vi "Application_CreateUninstallerBat.vi"(7 "TemporaryBatLocation":T1 items=["User Home"=0, "User Desktop"=1, "User Documents"=2, "User Application Data"=3, "User Preferences"=4, "User Temporary"=5, "Public Documents"=6, "Public Application Data"=7, "Public Preferences"=8, "Public Cache"=13, "System Core Libraries"=9, "System Installed Libraries"=10, "Application Files"=11, "Boot Volume Root"=12], 8 "error in":errorcluster, 11 "Project Name":string="BioReactor.lvproj") -> (0 "error IO":errorcluster)   [LabVIEW 2016]
doc: "Creates a windows .bat file with a time delay which is going to restart the project.\n\nAndreas Elmiger, 16.01.2017"
uses:
  <vilib>/Utility/sysdir.llb/System Directory Type.ctl
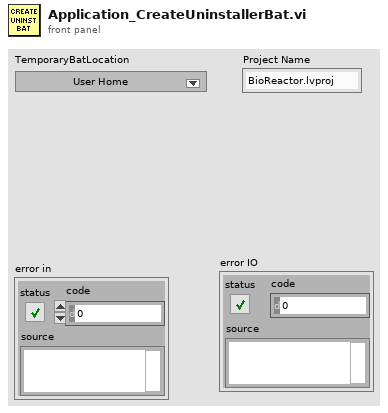
[diagram p1: front panel]
types:
  T1 = typedef "System Directory Type.ctl" = i32
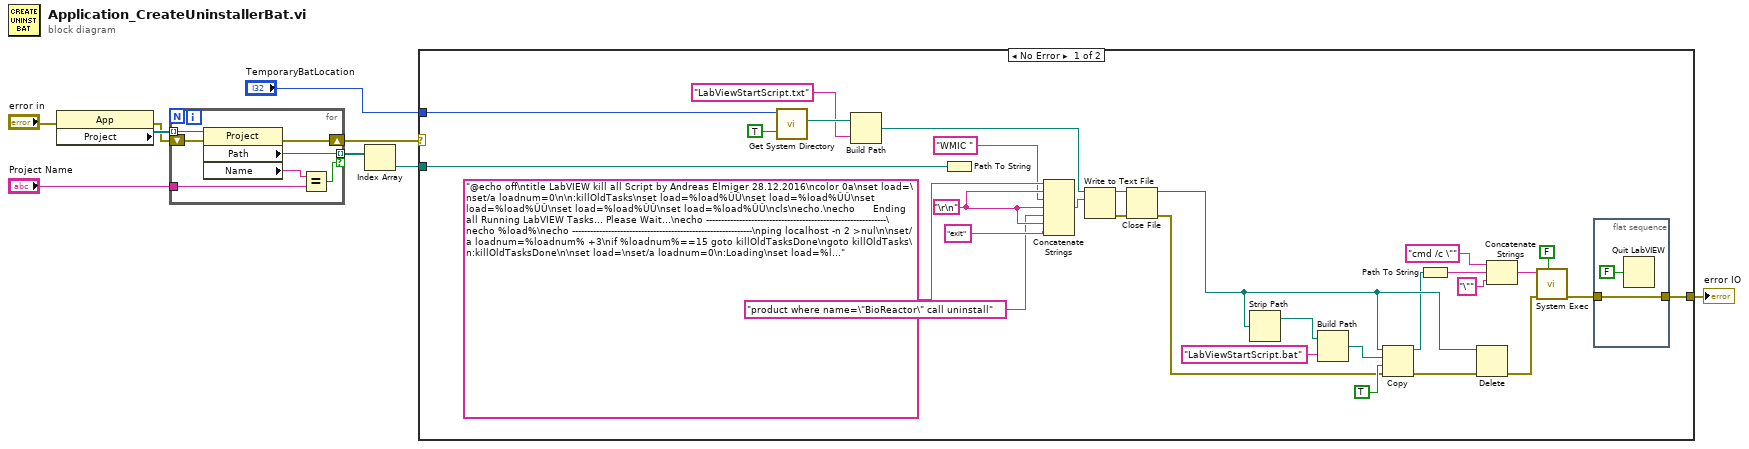
[diagram p0: block diagram]
diagram:
  n1 = property class="App"(error in="error in") -> (error out=w2:errorcluster, "Project"=w7:refnum<vi>[])  [unwired: 1 in, 1 out]
  n2 = for {
    tunnel: w7 -> [w16] mode=indexing
    tunnel: [w15] -> w5 mode=indexing if=w12
    tunnel: "Project Name" -> [w13]
    shift-right: [w10] -> w1
    shift-left: w2 -> [w11]
    n3 = property class="Project"(reference=w16, error in=w11) -> (error out=w10:errorcluster, "Path"=w15:path, "Name"=w14:string)  [unwired: 1 out]
    n4 = Equal?(x=w14, y=w13) -> (x = y?=w12:bool)
  }
  n5 = Index Array(array=w5) -> (element=w4:path)  [unwired: 1 in]
  n6 = case shown="No Error" w1 {
    selector: w1 -> [_ w49]
    tunnel: "TemporaryBatLocation" -> [w46 _]
    tunnel: w4 -> [w28 _]
    tunnel: [w21 w49] -> w8
    frame No Error {
      w20 = "\r\n"
      n7 = call <vilib>:"Get System Directory.vi"("create directory if not found? (F)"=TRUE, "system directory type"=w46) -> ("system directory"=w45:path)  [unwired: 9 in]
      n8 = Build Path(base path=w45, name or relative path="LabViewStartScript.txt" ("prompt (Choose or enter file path)")) -> (appended path=w38:path)
      n9 = Path To String(path=w28) -> ()  [unwired: 1 out]
      n10 = Concatenate Strings("@echo off\ntitle LabVIEW kill all Script by Andreas Elmiger 28.12.2016\ncolor 0a\nset load=\nset/a loadnum=0\n\n:killOldTasks\nset load=%load%ÛÛ\nset load=%load%ÛÛ\nset load=%load%ÛÛ\nset load=%load%ÛÛ\nset load=%load%ÛÛ\ncls\necho.\necho      Ending all Running LabVIEW Tasks... Please Wait...\necho ------------------------------------------------------------\necho %load%\necho ------------------------------------------------------------\nping localhost -n 2 >nul\n\nset/a loadnum=%loadnum% +3\nif %loadnum%==15 goto killOldTasksDone\ngoto killOldTasks\n:killOldTasksDone\n\nset load=\nset/a loadnum=0\n:Loading\nset load=%load%ÛÛ\nset load=%load%ÛÛ\nset load=%load%ÛÛ\nset load=%load%ÛÛ\nset load=%load%ÛÛ\ncls\necho.\necho         Loading LabVIEW Software... Please Wait...\necho ------------------------------------------------------------\necho %load%\necho ------------------------------------------------------------\nping localhost -n 2 >nul\n\nset/a loadnum=%loadnum% +3\nif %loadnum%==15 goto Done\n\ngoto Loading\n:Done" ("text"), w20, "WMIC " ("string"), w20, "product where name=\"BioReactor\" call uninstall" ("string"), w20, "exit" ("string")) -> (w27:string)
      n11 = Write to Text File(file (use dialog)=w38, text=w27) -> (refnum out=w43:refnum<file>, error out=w26:errorcluster)  [unwired: 2 in, 1 out]
      n12 = Close File(refnum=w43, error in=w26) -> (path=w32:path, error out=w25:errorcluster)
      n13 = Strip Path(path=w32) -> (stripped path=w36:path)  [unwired: 1 out]
      n14 = Build Path(base path=w36, name or relative path="LabViewStartScript.bat") -> (appended path=w35:path)
      n15 = Copy(8:w25, 9:TRUE ("overwrite (F)"), 10:w35, 11:w32) -> (0:w33:errorcluster, 3:w31:path)  [unwired: 1 in, 1 out]
      n16 = Path To String(path=w31) -> (string=w40:string)
      n17 = Delete(path (use dialog)=w32, error in=w33) -> (error out=w23:errorcluster)  [unwired: 3 in, 2 out]
      n18 = Concatenate Strings("cmd /c \"" ("command line"), w40, "\"" ("string")) -> (w41:string)
      n19 = call <vilib>:"System Exec.vi"("wait until completion? (T)"=FALSE, "error in (no error)"=w23, "command line"=w41) -> ("error out"=w22:errorcluster)  [unwired: 5 in, 3 out]
      n20 = flat-sequence {
        tunnel: w22 -> [w47]
        tunnel: [w47] -> w21
        frame #0 {
          n21 = Quit LabVIEW(quit? (T)=FALSE) -> ()
        }
      }
    }
    frame Error {
    }
  }
  "error IO" <- w8
